vi "PID_calc_Fi_corr.vi"(4 "Kd/Tau":fxp<+/-,32,4>, 5 "Ki*Tau":fxp<+/-,32,4>, 6 "Kp":fxp<+/-,32,4>, 7 "Reset":bool=TRUE, 8 "input valid":bool=TRUE, 9 "Fi_delta":fxp<+/-,32,4>, 10 "Fi_start":fxp<+/-,32,4>, 11 "Data in":fxp<+/-,16,14>[](array[numeric])=[0.0, 0.0, 0.0, 0.0]) -> (0 "output valid":bool, 2 "cos_fi_korr":fxp<+/-,16,2>, 3 "sin fi_korr":fxp<+/-,16,2>)   [LabVIEW 2013]
uses:
  <vilib>/rvi/FXPMathLib/FxpSinAndCos/subVIs/nifxpmath_SinAndCos_SimConfig.ctl
  <vilib>/rvi/FXPMathLib/FxpSinAndCos/simVIs/DllFxpSinAndCosTemp_sub.vi
  <vilib>/rvi/FXPMathLib/FxpSub/XNode/nifxpmath_Sub.xnode
  <vilib>/rvi/FXPMathLib/FxpAdd/XNode/nifxpmath_Add.xnode
  <vilib>/rvi/FXPMathLib/FxpSinAndCos/XNode/nifxpmath_SinAndCos.xnode
  <vilib>/rvi/FXPMathLib/FxpMul/XNode/nifxpmath_Multiplier.xnode
  <vilib>/rvi/FXPMathLib/sim/FxpSim.dll
panel:
  # "2*Pi*Fc*T_delay"
  # "2*Pi*Fc*delta_fi_increase"
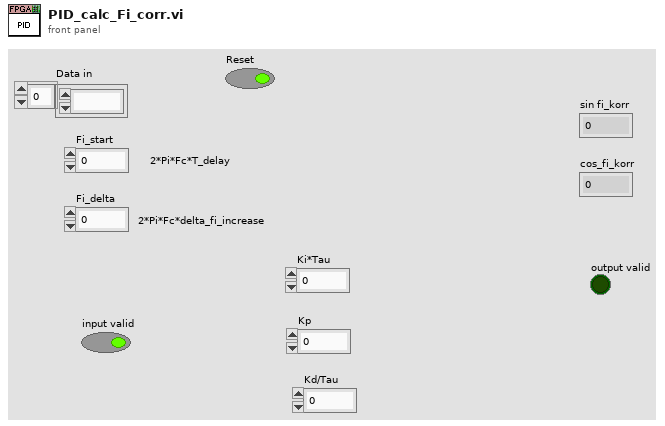
[diagram p1: front panel]
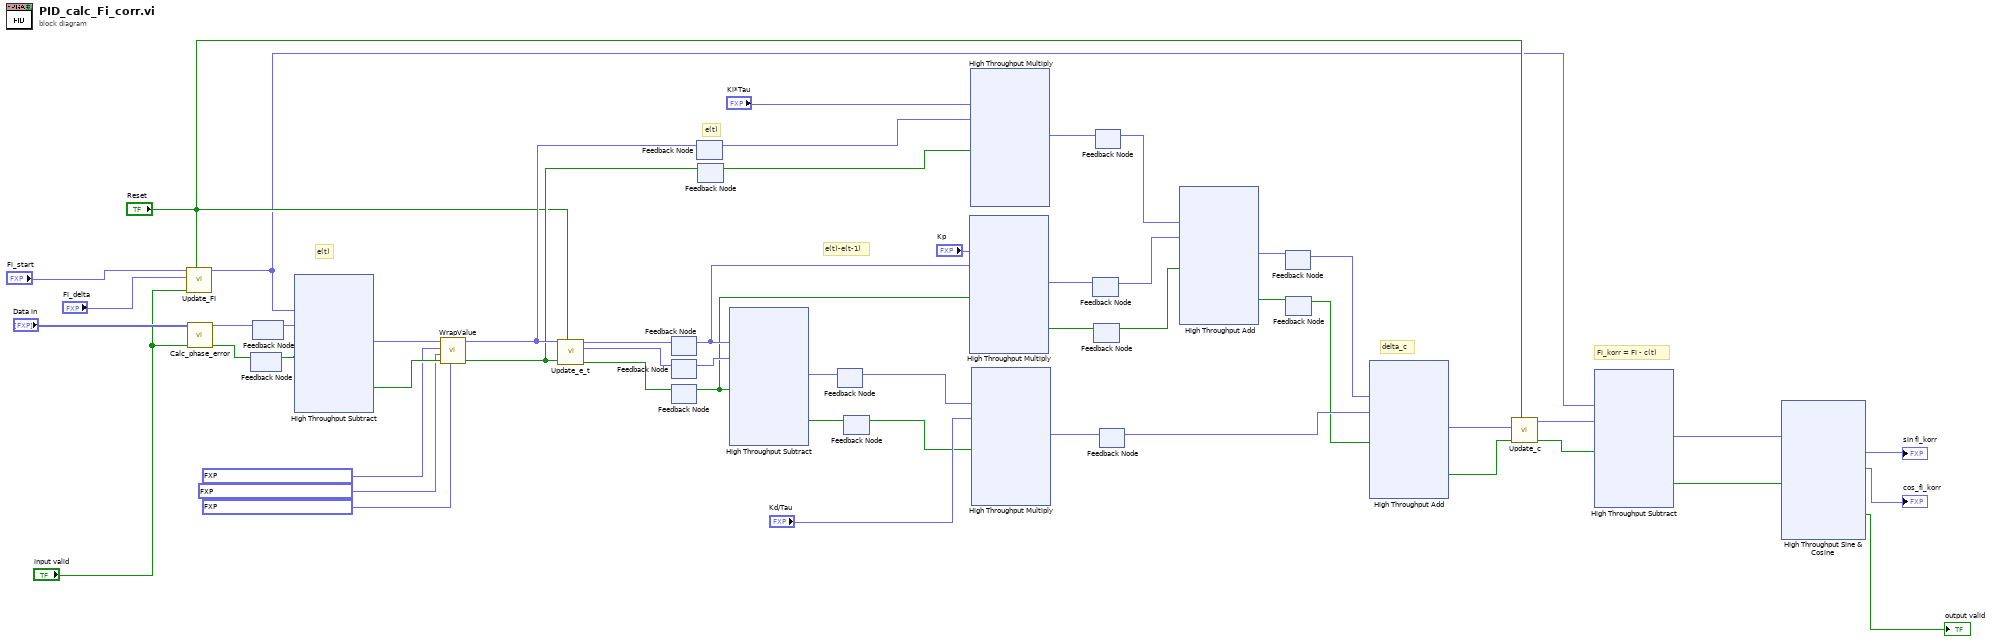
[diagram p0: block diagram]
diagram:
  # "Fi_korr = Fi - c(t)"
  # "delta_c"
  # "e(t)-e(t-1)"
  # "e(t)"
  # "e(t)"
  n1 = call "Update_FI.vi"("Reset"="Reset", "input valid"="input valid", "Fi_delta"="Fi_delta", "Fi_start"="Fi_start") -> ("Fi out"=w1:fxp<+/-,32,4>)  [unwired: 6 in, 1 out]
  n2 = call "Calc_phase_error.vi"("input valid"="input valid", "Data in"="Data in") -> ("output valid"=w47:bool, "Phase error"=w48:fxp<+/-,32,4>)  [unwired: 8 in]
  n3 = feedback #1() -> (w46:bool)  [unwired: 1 in]
  n4 = feedback-in #1(w47) -> ()
  n5 = feedback #2() -> (w51:fxp<+/-,32,4>)  [unwired: 1 in]
  n6 = feedback-in #2(w48) -> ()
  n7 = xnode "High Throughput Subtract"("x"=w1, "y"=w51, "input valid"=w46) -> ("x-y"=w34:fxp<+/-,32,4>, "output valid"=w33:bool)  [unwired: 1 in, 1 out]
  n8 = call "WrapValue.vi"("wrap_range"=fxp<+/-,32,4> 6.2831853069365025 ("wrap_max"), "Input valid"=w33, "wrap_min"=fxp<+/-,32,4> -3.1415926553308964 ("wrap_max"), "wrap_max"=fxp<+/-,32,4> 3.1415926553308964, "x_in"=w34) -> ("output valid"=w26:bool, "x_out"=w32:fxp<+/-,32,4>)  [unwired: 5 in]
  n9 = call "Update_e_t.vi"("Rest"="Reset", "input valid"=w26, "e(t)"=w32) -> ("output valid"=w43:bool, "e(t-1)-e(t-2)"=w44:fxp<+/-,32,4>, "e(t)-e(t-1)"=w45:fxp<+/-,32,4>)  [unwired: 6 in]
  n10 = feedback #3() -> (w27:fxp<+/-,32,4>)  [unwired: 1 in]
  n11 = feedback-in #3(w45) -> ()
  n12 = feedback #4() -> (w42:fxp<+/-,32,4>)  [unwired: 1 in]
  n13 = feedback-in #4(w44) -> ()
  n14 = feedback #5() -> (w25:bool)  [unwired: 1 in]
  n15 = feedback-in #5(w43) -> ()
  n16 = feedback #6() -> (w36:fxp<+/-,32,4>)  [unwired: 1 in]
  n17 = feedback-in #6(w32) -> ()
  n18 = feedback #7() -> (w24:bool)  [unwired: 1 in]
  n19 = feedback-in #7(w26) -> ()
  n20 = xnode "High Throughput Subtract"("x"=w27, "y"=w42, "input valid"=w25) -> ("x-y"=w40:fxp<+/-,32,4>, "output valid"=w39:bool)  [unwired: 1 in, 1 out]
  n21 = feedback #8() -> (w38:fxp<+/-,32,4>)  [unwired: 1 in]
  n22 = feedback-in #8(w40) -> ()
  n23 = feedback #9() -> (w28:bool)  [unwired: 1 in]
  n24 = feedback-in #9(w39) -> ()
  n25 = xnode ("High Throughput Multiply")("x"="Kp", "y"=w27, "input valid"=w25) -> ("x*y"=w21:fxp<+/-,32,4>, "output valid"=w19:bool)  [unwired: 1 in, 1 out]
  n26 = xnode ("High Throughput Multiply")("x"="Ki*Tau", "y"=w36, "input valid"=w24) -> ("x*y"=w23:fxp<+/-,32,4>)  [unwired: 1 in, 2 out]
  n27 = xnode ("High Throughput Multiply")("x"=w38, "y"="Kd/Tau", "input valid"=w28) -> ("x*y"=w17:fxp<+/-,32,4>)  [unwired: 1 in, 2 out]
  n28 = feedback #10() -> (w20:fxp<+/-,32,4>)  [unwired: 1 in]
  n29 = feedback-in #10(w21) -> ()
  n30 = feedback #11() -> (w18:bool)  [unwired: 1 in]
  n31 = feedback-in #11(w19) -> ()
  n32 = feedback #12() -> (w22:fxp<+/-,32,4>)  [unwired: 1 in]
  n33 = feedback-in #12(w23) -> ()
  n34 = feedback #13() -> (w16:fxp<+/-,32,4>)  [unwired: 1 in]
  n35 = feedback-in #13(w17) -> ()
  n36 = xnode "High Throughput Add"("x"=w22, "y"=w20, "input valid"=w18) -> ("x+y"=w15:fxp<+/-,32,4>, "output valid"=w14:bool)  [unwired: 1 in, 1 out]
  n37 = feedback #14() -> (w13:fxp<+/-,32,4>)  [unwired: 1 in]
  n38 = feedback-in #14(w15) -> ()
  n39 = feedback #15() -> (w12:bool)  [unwired: 1 in]
  n40 = feedback-in #15(w14) -> ()
  n41 = xnode "High Throughput Add"("x"=w13, "y"=w16, "input valid"=w12) -> ("x+y"=w11:fxp<+/-,32,4>, "output valid"=w10:bool)  [unwired: 1 in, 1 out]
  n42 = call "Update_c.vi"("Reset"="Reset", "input valid"=w10, "delta_c"=w11) -> ("output valid"=w7:bool, "c out"=w8:fxp<+/-,32,4>)  [unwired: 7 in]
  n43 = xnode "High Throughput Subtract"("x"=w1, "y"=w8, "input valid"=w7) -> ("x-y"=w6:fxp<+/-,32,4>, "output valid"=w3:bool)  [unwired: 1 in, 1 out]
  n44 = xnode "High Throughput Sine & Cosine"("x (pi)"=w6, "input valid"=w3) -> ("sin(x)"=→"sin fi_korr":fxp<+/-,16,2>, "cos(x)"=→"cos_fi_korr":fxp<+/-,16,2>, "output valid"=→"output valid":bool)  [unwired: 1 in, 1 out]
